vi "niFGEN - 1 Session Unregistered.vi"(8 "error in":errorcluster) -> (0 "error out":errorcluster, 3 "Session Reservation out":refnum<class "Session Reservation.lvclass">)   [LabVIEW 2020, in "MeasurementServerTests.lvlib"]
uses:
  MeasurementServerTests.lvlib
  Runtime/MeasurementLink Session Management/Session Reservation/Session Reservation.lvclass
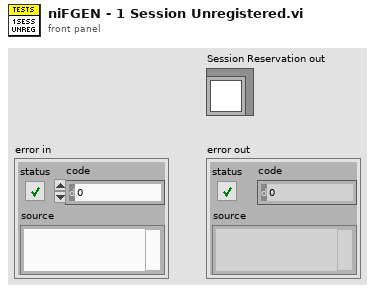
[diagram p1: front panel]
types:
  T1 = typedef "MeasurementLink Session Management.lvlib/Session Reservation.lvclass/Data.ctl" = cluster{"session and driver infos":T2[], "pin or relay names":string[], "connection map":refnum<class "Connection Map.lvclass">, "pin map context":T6, "reservation observer":refnum<class "IReservationObserver.lvclass">, "dvr valid":bool}
  T2 = typedef "MeasurementLink Session Management.lvlib/Session Reservation.lvclass/Session and Driver Info.ctl" = cluster{"session info":T3, "session":variant, "instrument":refnum<class "IInstrument.lvclass">}
  T3 = typedef "MeasurementLink Session Management Client.lvlib/ni_measurementlink_sessionmanagement_v1_SessionInformation.ctl" = cluster{"session":T4, "resource_name":string, "channel_list":string, "instrument_type_id":string, "session_exists":bool, "channel_mappings":T5[]}
  T4 = typedef "MeasurementLink Session Management Client.lvlib/nidevice_grpc_Session.ctl" = cluster{"name":string}
  T5 = typedef "MeasurementLink Session Management Client.lvlib/ni_measurementlink_sessionmanagement_v1_ChannelMapping.ctl" = cluster{"pin_or_relay_name":string, "site":i32, "channel":string}
  T6 = typedef "MeasurementLink Session Management Client.lvlib/ni_measurementlink_PinMapContext.ctl" = cluster{"pin_map_id":string, "sites":i32[]}
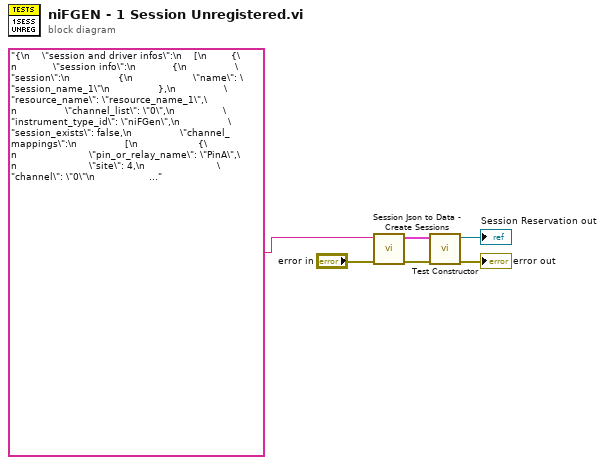
[diagram p0: block diagram]
diagram:
  n1 = call "Session Json to Data - Create Sessions.vi"("error in"="error in", "json in"="{\n    \"session and driver infos\":\n    [\n        {\n            \"session info\":\n            {\n                \"session\":\n                {\n                    \"name\": \"session_name_1\"\n                },\n                \"resource_name\": \"resource_name_1\",\n                \"channel_list\": \"0\",\n                \"instrument_type_id\": \"niFGen\",\n                \"session_exists\": false,\n                \"channel_mappings\":\n                [\n                    {\n                        \"pin_or_relay_name\": \"PinA\",\n                        \"site\": 4,\n                        \"channel\": \"0\"\n                    }\n                ]\n            }\n        }\n    ],\n    \"dvr valid\": true\n}") -> ("error out"=w3:errorcluster, "data out"=w2:T1)  [unwired: 8 in]
  n2 = call "Test Constructor.vi"("error in"=w3, "data"=w2) -> ("error out"=→"error out":errorcluster, "Session Reservation out"=→"Session Reservation out":refnum<class "Session Reservation.lvclass">)  [unwired: 8 in]
